vi "Get System Date & TIme.vi"(7 "want seconds? (F)":bool, 11 "date format (0)":enum16{"short", "long", "abbreviated"}(ring)) -> (3 "Current System Date & Time":T1)   [LabVIEW 2021]
uses:
  Controls/Current System Date & Time.ctl
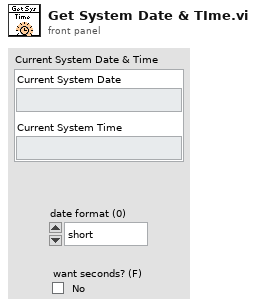
[diagram p1: front panel]
types:
  T1 = typedef "Current System Date & Time.ctl" = cluster{"Current System Time":string, "Current System Date":string}
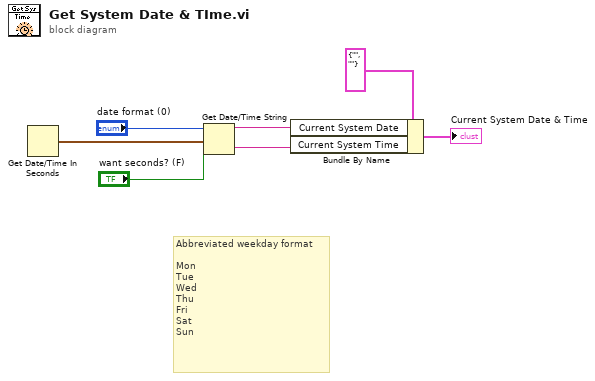
[diagram p0: block diagram]
diagram:
  # "Abbreviated weekday format\n\nMon\nTue\nWed\nThu\nFri\nSat\nSun"
  n1 = Get Date/Time In Seconds() -> (seconds since 1Jan1904=w1:timestamp)
  n2 = Get Date/Time String(date format (0)="date format (0)", seconds (now)=w1, want seconds? (F)="want seconds? (F)") -> (date string=w7:string, time string=w6:string)
  n3 = Bundle By Name(cluster=T1 {"Current System Time"="", "Current System Date"=""} ("Current System Date & Time"), "Current System Date"=w7, "Current System Time"=w6) -> (→"Current System Date & Time":T1)
